vi "Complete_V1.vi"() -> ()   [LabVIEW 2022 SP3]
uses:
  3bc9a862-b596-42d5-8eeb-dbbdc4778f0e.vi
  c1c20892-292a-4efc-bbee-37fc852e39ed.vi
  9a851694-c6f2-4fb5-8eff-591639fa9214.vi
  <vilib>/Instr/_visa.llb/VISA Configure Serial Port (Instr).vi
  <vilib>/Utility/inputDevices.llb/keyboardAcquire.vi
panel:
  in  "Adj Parameter Value":string
  in  "Adj Set Parameter":string(combo)
  in  "Set Adjuster":bool
  in  "AutoScroll":bool
  in  "Ping Current Adjuster":bool
  out "Up":bool
  out "Down":bool
  out "Right":bool
  out "Left":bool
  out "Controller Feedback":string
  out "Controller Get Command Sent":string
  in  "Controller Info to Get":string(combo)
  in  "Get Controller Information":bool
  out "Adj Get Command Sent":string
  in  "Adjuster Info to Get":string(combo)
  in  "Print All Adjuster Positions":bool
  in  "Get Current Adj Information":bool
  out "Power Command Sent":string
  in  "POWER TO SYSTEM":bool
  in  "Run to end -Y":bool
  in  "Run to end +Y":bool
  in  "Run to end -X":bool
  in  "Run to end +X":bool
  in  "VISA Resource Name":refnum<visa-resource-name>
  in  "Adjustor Number":dbl format="%0#3_4p"
  in  "Emergency Stop":bool
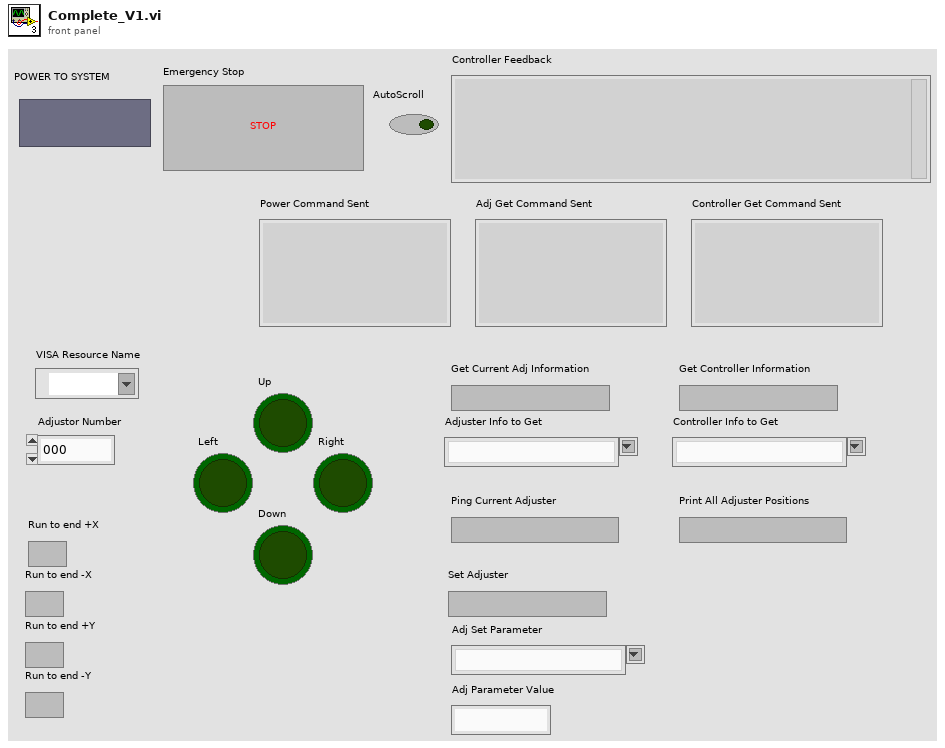
[diagram p1: front panel]
types:
  T1 = enum16{"0", "1", "2", "3", "4", "5", "6", "7", "8", "9", "A", "B", "C", "D", "E", "F", "G", "H", "I", "J", "K", "L", "M", "N", "O", "P", "Q", "R", "S", "T", "U", "V", "W", "X", "Y", "Z", "F1", "F2", "F3", "F4", "F5", "F6", "F7", "F8", "F9", "F10", "F11", "F12", "F13", "F14", "F15", "ADD", "BACK", "BACKSLASH", "CAPITAL", "COMMA", "DECIMAL", "DELETE", "DIVIDE", "DOWN", "END", "EQUALS", "ESCAPE", "GRAVE (`)", "HOME", "INSERT", "LBRACKET", "LCONTROL", "LEFT", "L ALT", "LSHIFT", "LWIN", "MINUS", "MULTIPLY", "NEXT", "NUMLOCK", "NUMPAD_0", "NUMPAD_1", "NUMPAD_2", "NUMPAD_3", "NUMPAD_4", "NUMPAD_5", "NUMPAD_6", "NUMPAD_7", "NUMPAD_8", "NUMPAD_9", "PAUSE", "PERIOD", "PRIOR (PG UP)", "RBRACKET", "RCONTROL", "RETURN", "RIGHT", "R ALT", "RSHIFT", "RWIN", "SCROLL", "SEMICOLON", "SLASH", "SPACE", "SUBTRACT", "TAB", "UP", "ENTER (num pad)", "' (quote)"}
  T2 = enum16{"0", "1", "2", "3", "4", "5", "6", "7", "8", "9", "A", "B", "C", "D", "E", "F", "G", "H", "I", "J", "K", "L", "M", "N", "O", "P", "Q", "R", "S", "T", "U", "V", "W", "X", "Y", "Z", "F1", "F2", "F3", "F4", "F5", "F6", "F7", "F8", "F9", "F10", "F11", "F12", "F13", "F14", "F15", "ADD", "BACK", "BACKSLASH", "CAPITAL", "COMMA", "DECIMAL", "DELETE", "DIVIDE", "DOWN", "END", "EQUALS", "ESCAPE", "GRAVE (`)", "HOME", "INSERT", "LBRACKET", "LCONTROL", "LEFT", "L ALT", "LSHIFT", "LWIN", "MINUS", "MULTIPLY", "NEXT", "NUMLOCK", "NUMPAD_0", "NUMPAD_1", "NUMPAD_2", "NUMPAD_3", "NUMPAD_4", "NUMPAD_5", "NUMPAD_6", "NUMPAD_7", "NUMPAD_8", "NUMPAD_9", "PAUSE", "PERIOD", "PRIOR (PG UP)", "RBRACKET", "RCONTROL", "RETURN", "RIGHT", "R ALT", "RSHIFT", "RWIN", "SCROLL", "SEMICOLON", "SLASH", "SPACE", "SUBTRACT", "TAB", "UP", "ENTER (num pad)", "' (quote)"}[]
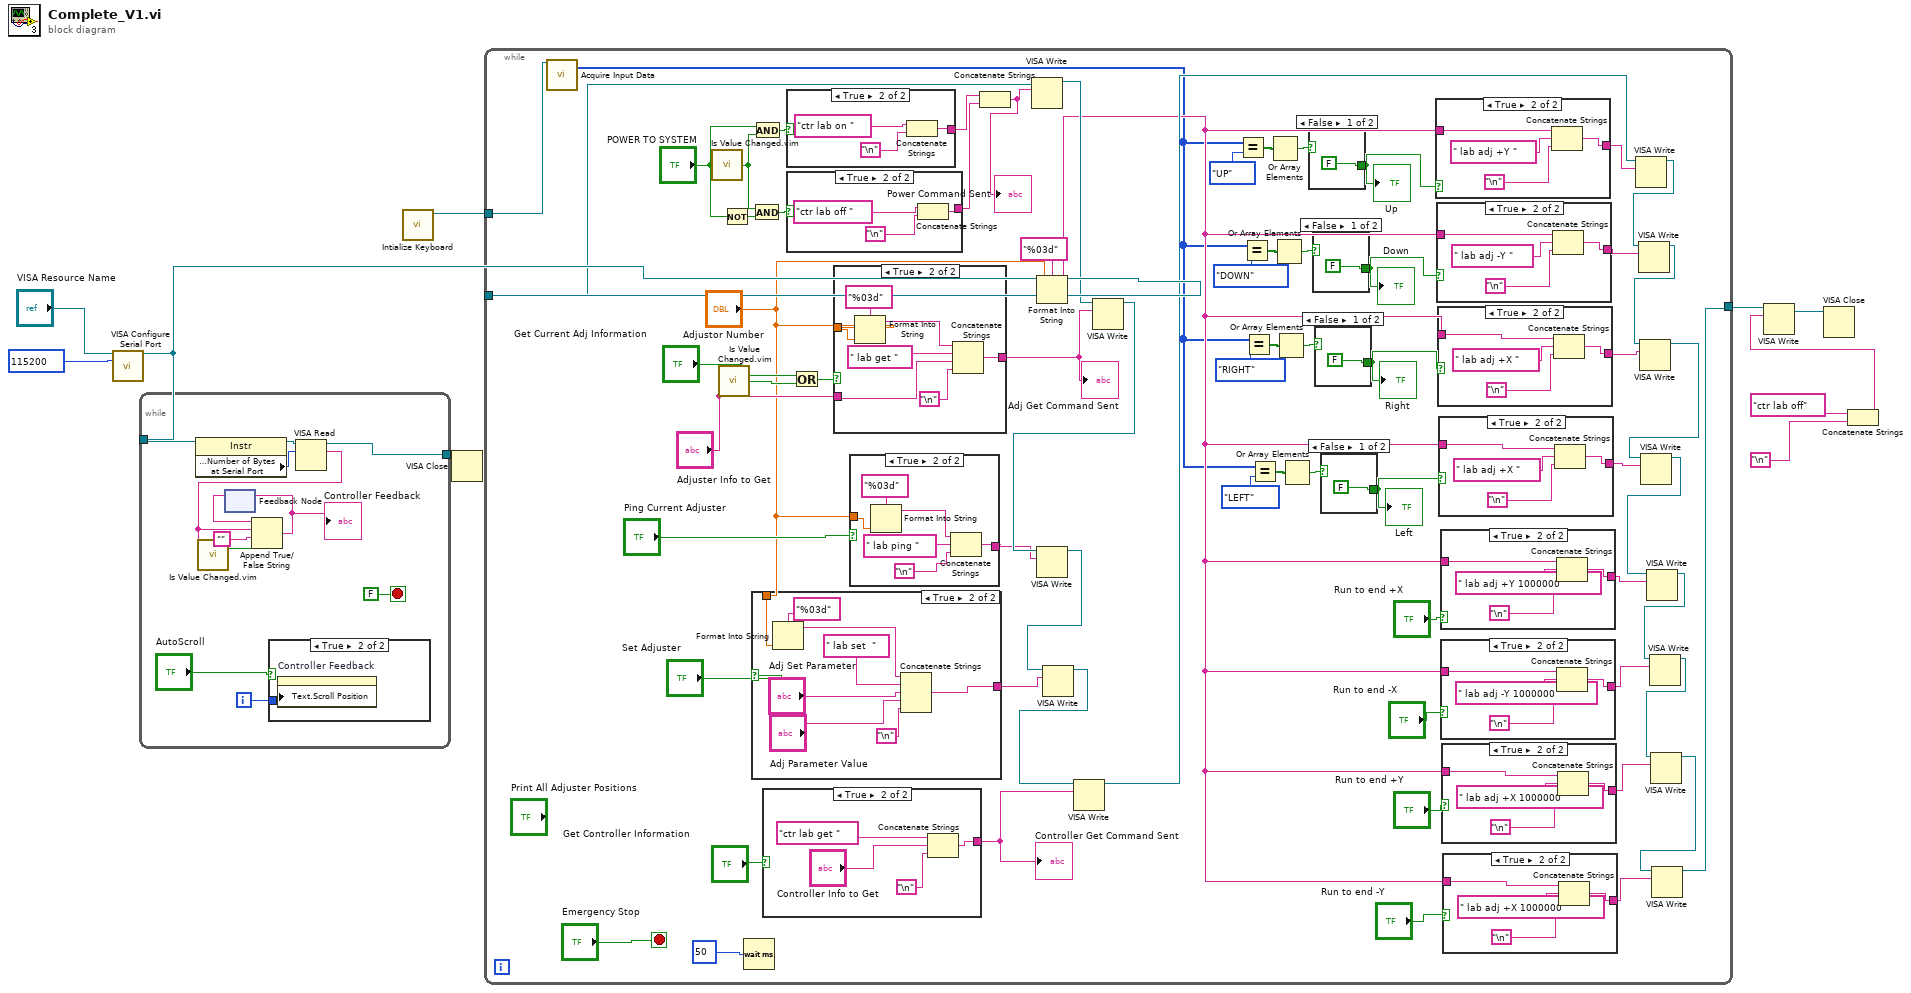
[diagram p0: block diagram]
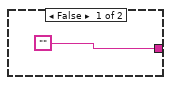
[diagram p3: hidden frame]
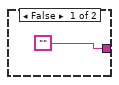
[diagram p4: hidden frame]
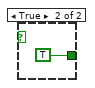
[diagram p5: hidden frame]
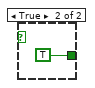
[diagram p6: hidden frame]
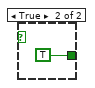
[diagram p7: hidden frame]
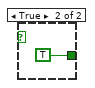
[diagram p8: hidden frame]
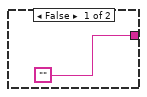
[diagram p9: hidden frame]
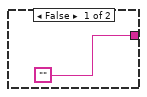
[diagram p10: hidden frame]
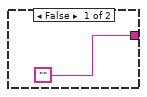
[diagram p11: hidden frame]
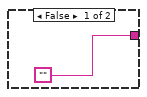
[diagram p12: hidden frame]
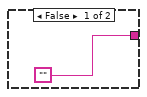
[diagram p13: hidden frame]
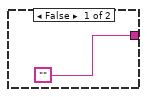
[diagram p14: hidden frame]
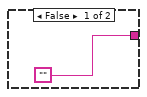
[diagram p15: hidden frame]
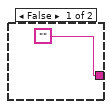
[diagram p16: hidden frame]
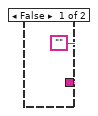
[diagram p17: hidden frame]
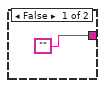
[diagram p18: hidden frame]
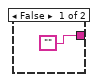
[diagram p19: hidden frame]
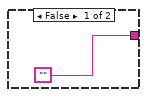
[diagram p20: hidden frame]
diagram:
  n1 = call-poly "VISA Configure Serial Port"("VISA resource name"="VISA Resource Name", "baud rate (9600)"=u32 115200) -> ("VISA resource name out"=w3:refnum<visa-resource-name>)  [unwired: 12 in, 1 out]
  n2 = while {
    tunnel: w3 -> [w15]
    tunnel: [w14] -> w2
    i -> [w12]
    stop <- FALSE stop-if-true
    n3 = property class="Instr"(reference=w15) -> (reference out=w22:refnum<visa-resource-name>, "Serial Settings:Number of Bytes at Serial Port"=w21:u32)  [unwired: 1 in, 1 out]
    n4 = feedback #1() -> (w18:string)  [unwired: 1 in]
    n5 = case shown="True" "AutoScroll" {
      tunnel: w12 -> [_ w23]
      frame False {
      }
      frame True {
        n6 = property on="Controller Feedback" class="Str"("Text.Scroll Position"=w23) -> ()  [unwired: 2 in, 2 out]
      }
    }
    n7 = VISA Read(VISA resource name=w22, byte count=w21) -> (VISA resource name out=w14:refnum<visa-resource-name>, read buffer=w19:string)  [unwired: 1 in, 2 out]
    n8 = call "Is Value Changed.vim"("value"=w19) -> ("changed or first call?"=w20:bool)
    n9 = Append True/False String(1:w20, 2:"", 3:w19, 4:w18) -> (0:w16:string)
    "Controller Feedback" <- w16
    n10 = feedback-in #1(w16) -> ()
  }
  n11 = call <vilib>:"Intialize Keyboard.vi"() -> ("device ID"=w1:refnum<k1>)  [unwired: 10 in, 1 out]
  n12 = VISA Close(VISA resource name=w2) -> ()  [unwired: 1 in, 1 out]
  n13 = while {
    tunnel: w3 -> [w90]
    tunnel: [w57] -> w9
    tunnel: w1 -> [w53]
    stop <- "Emergency Stop" stop-if-true
    n14 = call-poly <vilib>:"Acquire Input Data.vi"("device ID"=w53) -> ("keys pressed"=w36:T2)  [unwired: 16 in, 2 out]
    n15 = call "Is Value Changed.vim"("value"="POWER TO SYSTEM") -> ("changed or first call?"=w83:bool)
    n16 = call "Is Value Changed.vim"("value"="Adjuster Info to Get") -> ("changed or first call?"=w30:bool)
    n17 = Not(x="POWER TO SYSTEM") -> (.not. x?=w88:bool)
    n18 = Wait (ms)(milliseconds to wait=50) -> ()  [unwired: 1 out]
    n19 = And(x=w83, y=w88) -> (x .and. y?=w87:bool)
    n20 = case shown="True" "Set Adjuster" {
      tunnel: ["" w98] -> w25
      tunnel: "Adjustor Number" -> [_ w96]
      frame False {
      }
      frame True {
        n21 = Format Into String(format string="%03d", w96) -> (resulting string=w97:string)  [unwired: 2 in, 1 out]
        n22 = Concatenate Strings(w97, " lab set  ", "Adj Set Parameter", "Adj Parameter Value", "\n") -> (w98:string)
      }
    }
    n23 = And(x="POWER TO SYSTEM", y=w83) -> (x .and. y?=w89:bool)
    n24 = case shown="True" "Get Controller Information" {
      tunnel: ["" w152] -> w78
      frame False {
      }
      frame True {
        n25 = Concatenate Strings("ctr lab get ", "Controller Info to Get", "\n") -> (w152:string)
      }
    }
    "Controller Get Command Sent" <- w78
    n26 = case shown="True" w89 {
      tunnel: ["" w170] -> w86
      frame False {
      }
      frame True {
        n27 = Concatenate Strings("ctr lab on ", "\n") -> (w170:string)
      }
    }
    n28 = case shown="True" w87 {
      tunnel: ["" w166] -> w85
      frame False {
      }
      frame True {
        n29 = Concatenate Strings("ctr lab off ", "\n") -> (w166:string)
      }
    }
    n30 = Or(x="Get Current Adj Information", y=w30) -> (x .or. y?=w29:bool)
    n31 = case shown="True" w29 {
      tunnel: "Adjustor Number" -> [_ w160]
      tunnel: ["" w159] -> w80
      tunnel: "Adjuster Info to Get" -> [_ w157]
      frame False {
      }
      frame True {
        n32 = Format Into String(format string="%03d", w160) -> (resulting string=w158:string)  [unwired: 2 in, 1 out]
        n33 = Concatenate Strings(w158, " lab get ", w157, "\n") -> (w159:string)
      }
    }
    "Adj Get Command Sent" <- w80
    n34 = case shown="True" "Ping Current Adjuster" {
      tunnel: "Adjustor Number" -> [_ w105]
      tunnel: ["" w104] -> w33
      frame False {
      }
      frame True {
        n35 = Format Into String(format string="%03d", w105) -> (resulting string=w103:string)  [unwired: 2 in, 1 out]
        n36 = Concatenate Strings(w103, " lab ping ", "\n") -> (w104:string)
      }
    }
    n37 = Concatenate Strings(w86, w85) -> (w82:string)
    "Power Command Sent" <- w82
    n38 = VISA Write(VISA resource name=w90, write buffer=w82) -> (VISA resource name out=w81:refnum<visa-resource-name>)  [unwired: 1 in, 2 out]
    n39 = Format Into String(format string="%03d", "Adjustor Number") -> (resulting string=w55:string)  [unwired: 2 in, 1 out]
    n40 = VISA Write(VISA resource name=w81, write buffer=w80) -> (VISA resource name out=w34:refnum<visa-resource-name>)  [unwired: 1 in, 2 out]
    n41 = VISA Write(VISA resource name=w34, write buffer=w33) -> (VISA resource name out=w26:refnum<visa-resource-name>)  [unwired: 1 in, 2 out]
    n42 = VISA Write(VISA resource name=w26, write buffer=w25) -> (VISA resource name out=w24:refnum<visa-resource-name>)  [unwired: 1 in, 2 out]
    n43 = VISA Write(VISA resource name=w24, write buffer=w78) -> (VISA resource name out=w77:refnum<visa-resource-name>)  [unwired: 1 in, 2 out]
    n44 = Equal?(x=w36, y=T1."UP" ("keyType 3")) -> (x = y?=w39:bool[])
    n45 = Equal?(x=w36, y=T1."DOWN" ("keyType 3")) -> (x = y?=w43:bool[])
    n46 = Equal?(x=w36, y=T1."RIGHT" ("keyType 3")) -> (x = y?=w47:bool[])
    n47 = Equal?(x=w36, y=T1."LEFT" ("keyType 3")) -> (x = y?=w51:bool[])
    n48 = Or Array Elements(Boolean array=w39) -> (logical OR=w38:bool)
    n49 = Or Array Elements(Boolean array=w43) -> (logical OR=w42:bool)
    n50 = Or Array Elements(Boolean array=w47) -> (logical OR=w46:bool)
    n51 = Or Array Elements(Boolean array=w51) -> (logical OR=w50:bool)
    n52 = case shown="False" w38 {
      tunnel: [FALSE TRUE] -> w37
      frame False {
      }
      frame True {
      }
    }
    "Up" <- w37
    n53 = case shown="False" w42 {
      tunnel: [FALSE TRUE] -> w41
      frame False {
      }
      frame True {
      }
    }
    "Down" <- w41
    n54 = case shown="False" w46 {
      tunnel: [FALSE TRUE] -> w45
      frame False {
      }
      frame True {
      }
    }
    "Right" <- w45
    n55 = case shown="False" w50 {
      tunnel: [FALSE TRUE] -> w49
      frame False {
      }
      frame True {
      }
    }
    "Left" <- w49
    n56 = case shown="True" w37 {
      tunnel: ["" w173] -> w76
      tunnel: w55 -> [_ w176]
      frame False {
      }
      frame True {
        n57 = Concatenate Strings(w176, " lab adj +Y ", "\n") -> (w173:string)
      }
    }
    n58 = case shown="True" w41 {
      tunnel: ["" w147] -> w75
      tunnel: w55 -> [_ w150]
      frame False {
      }
      frame True {
        n59 = Concatenate Strings(w150, " lab adj -Y ", "\n") -> (w147:string)
      }
    }
    n60 = case shown="True" w45 {
      tunnel: ["" w142] -> w73
      tunnel: w55 -> [_ w145]
      frame False {
      }
      frame True {
        n61 = Concatenate Strings(w145, " lab adj +X ", "\n") -> (w142:string)
      }
    }
    n62 = case shown="True" w49 {
      tunnel: ["" w137] -> w71
      tunnel: w55 -> [_ w140]
      frame False {
      }
      frame True {
        n63 = Concatenate Strings(w140, " lab adj +X ", "\n") -> (w137:string)
      }
    }
    n64 = case shown="True" "Run to end +X" {
      tunnel: ["" w132] -> w65
      tunnel: w55 -> [_ w135]
      frame False {
      }
      frame True {
        n65 = Concatenate Strings(w135, " lab adj +Y 1000000 ", "\n") -> (w132:string)
      }
    }
    n66 = case shown="True" "Run to end -X" {
      tunnel: ["" w127] -> w62
      tunnel: w55 -> [_ w130]
      frame False {
      }
      frame True {
        n67 = Concatenate Strings(w130, " lab adj -Y 1000000 ", "\n") -> (w127:string)
      }
    }
    n68 = case shown="True" "Run to end +Y" {
      tunnel: ["" w122] -> w60
      tunnel: w55 -> [_ w125]
      frame False {
      }
      frame True {
        n69 = Concatenate Strings(w125, " lab adj +X 1000000 ", "\n") -> (w122:string)
      }
    }
    n70 = case shown="True" "Run to end -Y" {
      tunnel: ["" w117] -> w58
      tunnel: w55 -> [_ w120]
      frame False {
      }
      frame True {
        n71 = Concatenate Strings(w120, " lab adj +X 1000000 ", "\n") -> (w117:string)
      }
    }
    n72 = VISA Write(VISA resource name=w77, write buffer=w76) -> (VISA resource name out=w74:refnum<visa-resource-name>)  [unwired: 1 in, 2 out]
    n73 = VISA Write(VISA resource name=w74, write buffer=w75) -> (VISA resource name out=w72:refnum<visa-resource-name>)  [unwired: 1 in, 2 out]
    n74 = VISA Write(VISA resource name=w72, write buffer=w73) -> (VISA resource name out=w70:refnum<visa-resource-name>)  [unwired: 1 in, 2 out]
    n75 = VISA Write(VISA resource name=w70, write buffer=w71) -> (VISA resource name out=w64:refnum<visa-resource-name>)  [unwired: 1 in, 2 out]
    n76 = VISA Write(VISA resource name=w64, write buffer=w65) -> (VISA resource name out=w63:refnum<visa-resource-name>)  [unwired: 1 in, 2 out]
    n77 = VISA Write(VISA resource name=w63, write buffer=w62) -> (VISA resource name out=w61:refnum<visa-resource-name>)  [unwired: 1 in, 2 out]
    n78 = VISA Write(VISA resource name=w61, write buffer=w60) -> (VISA resource name out=w59:refnum<visa-resource-name>)  [unwired: 1 in, 2 out]
    n79 = VISA Write(VISA resource name=w59, write buffer=w58) -> (VISA resource name out=w57:refnum<visa-resource-name>)  [unwired: 1 in, 2 out]
  }
  n80 = Concatenate Strings("ctr lab off", "\n") -> (w5:string)
  n81 = VISA Write(VISA resource name=w9, write buffer=w5) -> (VISA resource name out=w8:refnum<visa-resource-name>)  [unwired: 1 in, 2 out]
  n82 = VISA Close(VISA resource name=w8) -> ()  [unwired: 1 in, 1 out]
